vi "Add DAQ Hardware.vi"(7 "Overwrite Existing?":bool=TRUE, 8 "error in (no error)":errorcluster, 9 "Settings":T1={"Name"="", "Description"="", "InputConfiguration"=10078, "TurnOffHWTimedSinglePointAI"=FALSE, "TurnOffHWTimedSinglePointAO"=FALSE, "DAQConversionRateOption"=0, "PortWidth"=8, "Analog Inputs"=[], "Analog Outputs"=[], "DIO Port Settings"=[], "Counter Settings"={"Frequency Measurements"=[], "Period Measurements"=[], "Count Measurements"=[], "Position Measurements"=[]}} {"Counter Settings"."Position Measurements"."ZIndexMode" items=["AHighBHigh"=10040, "AHighBLow"=10041, "ALowBHigh"=10042, "ALowBLow"=10043]; "Counter Settings"."Position Measurements"."Decoding" items=["Decoding1X"=10090, "Decoding2X"=10091, "Decoding4X"=10092, "DecodingPulseCounting"=10313]; "Counter Settings"."Count Measurements"."CountDirection" items=["Down"=10124, "Up"=10128, "ExternallyControlled"=10326]; "Counter Settings"."Count Measurements"."Edge" items=["Falling"=10171, "Rising"=10280]; "Counter Settings"."Period Measurements"."Edge" items=["Falling"=10171, "Rising"=10280]; "Counter Settings"."Frequency Measurements"."Edge" items=["Falling"=10171, "Rising"=10280]; "Analog Outputs"."ChannelType" items=["Voltage", "Current"]; "Analog Inputs"."ChannelType" items=["Voltage", "Current"]; "DAQConversionRateOption" items=["Default", "Maximum"]; "InputConfiguration" items=["NRSE"=10078, "RSE"=10083, "Differential"=10106, "Pseudodifferential"=12529, "Default"=-1]}, 10 "Base Node Path":string="Targets/Controller/Hardware/Chassis/DAQ", 11 "SysDef Ref":T8) -> (0 "error out":errorcluster, 2 "New Node Path":string, 3 "SysDef Ref Out":T8)   [LabVIEW 2019, in "Simple SysDef API.lvlib"]
uses:
  <userlib>/SimpleSysDef/Simple SysDef API.lvlib
  <userlib>/SimpleSysDef/_SubVIs/System Definition Reference.ctl
  NationalInstruments.VeriStand.SystemDefinitionAPI
  <userlib>/SimpleSysDef/_SubVIs/Add DAQ Hardware_Settings.ctl
  <userlib>/SimpleSysDef/_SubVIs/Add DAQ Hardware_Analog Settings.ctl
  <userlib>/SimpleSysDef/_SubVIs/Add DAQ Hardware_Digital Port Settings.ctl
  <userlib>/SimpleSysDef/_SubVIs/Add DAQ Hardware_Digital Settings.ctl
  <userlib>/SimpleSysDef/_SubVIs/Add Frequency Measurement Channels_Settings.ctl
  <userlib>/SimpleSysDef/_SubVIs/Add Count Measurement Channels_Settings.ctl
  <userlib>/SimpleSysDef/_SubVIs/Add Position Measurement Channels_Settings.ctl
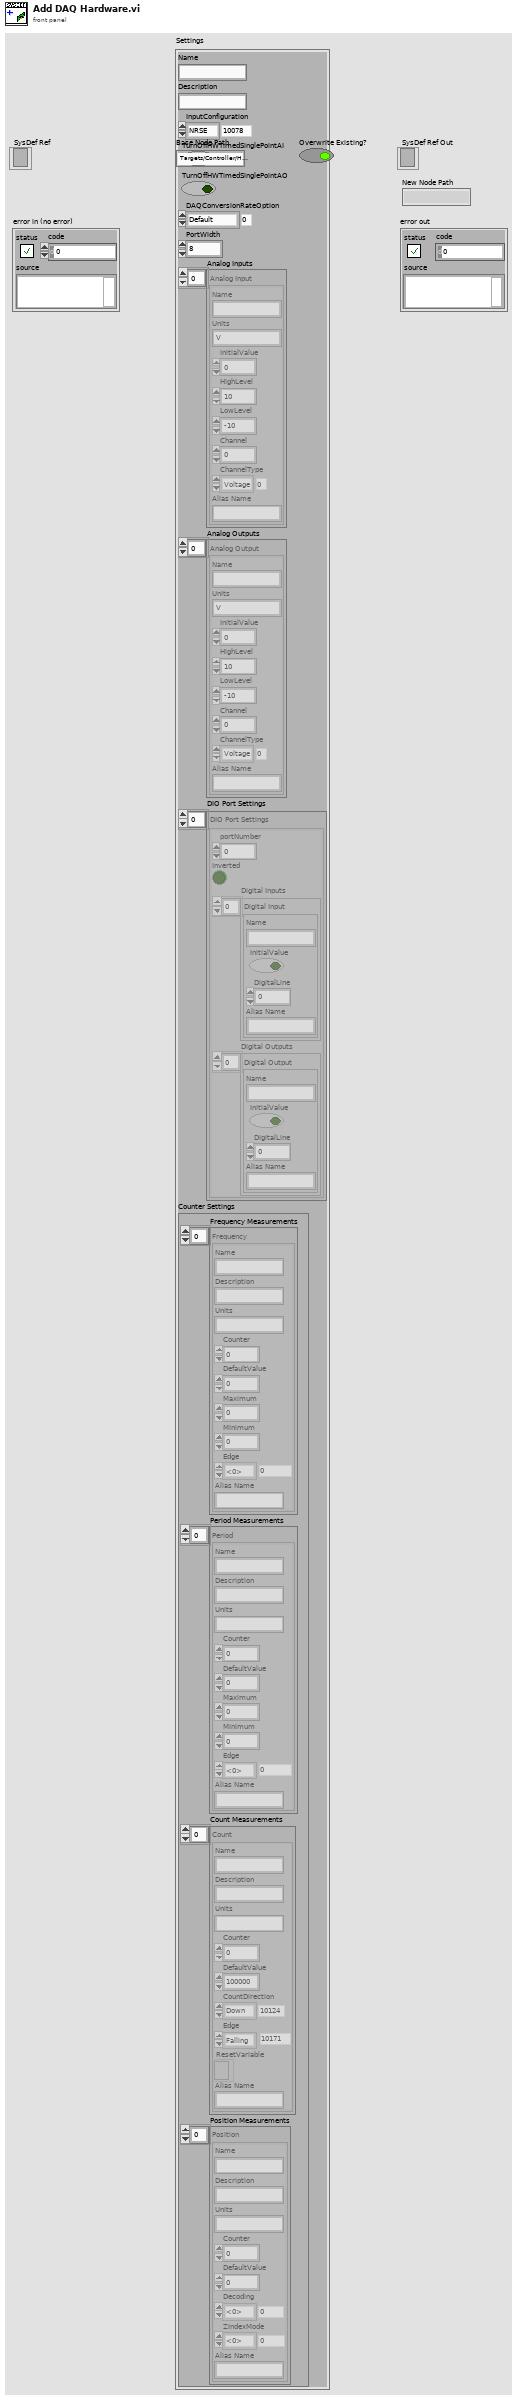
[diagram p1: front panel]
types:
  T1 = typedef "Simple SysDef API.lvlib/Add DAQ Hardware_Settings.ctl" = cluster{"Name":string, "Description":string, "InputConfiguration":i32, "TurnOffHWTimedSinglePointAI":bool, "TurnOffHWTimedSinglePointAO":bool, "DAQConversionRateOption":i32, "PortWidth":u16, "Analog Inputs":T2[], "Analog Outputs":T2[], "DIO Port Settings":T3[], "Counter Settings":cluster{"Frequency Measurements":T5[], "Period Measurements":T5[], "Count Measurements":T6[], "Position Measurements":T7[]}}
  T2 = typedef "Simple SysDef API.lvlib/Add DAQ Hardware_Analog Settings.ctl" = cluster{"Name":string, "Units":string, "InitialValue":dbl, "HighLevel":dbl, "LowLevel":dbl, "Channel":u32, "ChannelType":i32, "Alias Name":string}
  T3 = typedef "Simple SysDef API.lvlib/Add DAQ Hardware_Digital Port Settings.ctl" = cluster{"portNumber":u32, "Inverted":bool, "Digital Inputs":T4[], "Digital Outputs":T4[]}
  T4 = typedef "Simple SysDef API.lvlib/Add DAQ Hardware_Digital Settings.ctl" = cluster{"Name":string, "InitialValue":bool, "DigitalLine":u32, "Alias Name":string}
  T5 = typedef "Simple SysDef API.lvlib/Add Frequency Measurement Channels_Settings.ctl" = cluster{"Name":string, "Description":string, "Units":string, "Counter":u32, "DefaultValue":dbl, "Maximum":dbl, "Minimum":dbl, "Edge":i32, "Alias Name":string}
  T6 = typedef "Simple SysDef API.lvlib/Add Count Measurement Channels_Settings.ctl" = cluster{"Name":string, "Description":string, "Units":string, "Counter":u32, "DefaultValue":dbl, "CountDirection":i32, "Edge":i32, "ResetVariable":refnum<k24>, "Alias Name":string}
  T7 = typedef "Simple SysDef API.lvlib/Add Position Measurement Channels_Settings.ctl" = cluster{"Name":string, "Description":string, "Units":string, "Counter":u32, "DefaultValue":dbl, "Decoding":i32, "ZIndexMode":i32, "Alias Name":string}
  T8 = typedef "Simple SysDef API.lvlib/System Definition Reference.ctl" = refnum<k24>
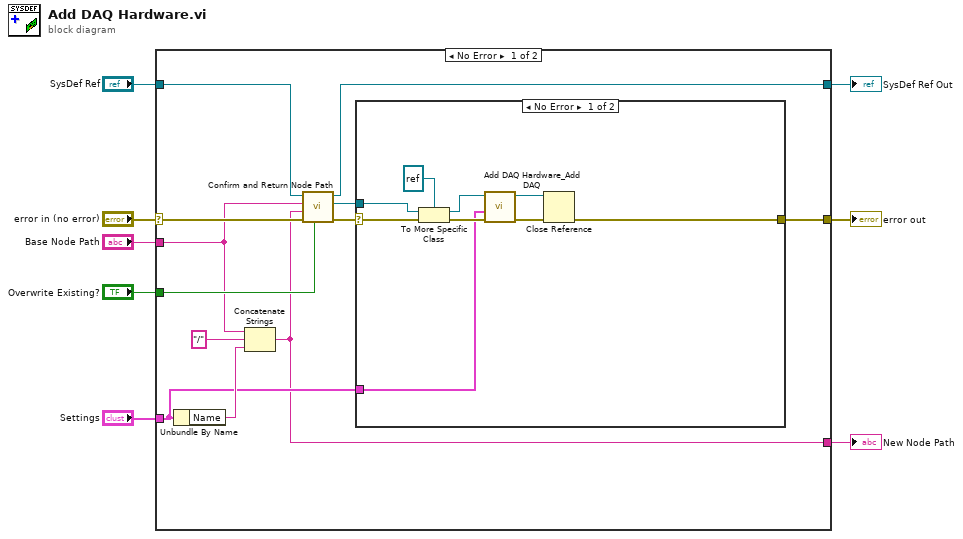
[diagram p0: block diagram]
diagram:
  n1 = case shown="No Error" "error in (no error)" {
    selector: "error in (no error)" -> [w20 w32]
    tunnel: [w16 w32] -> w7
    tunnel: "SysDef Ref" -> [w19 w31]
    tunnel: [w9 w31] -> w5
    tunnel: "Base Node Path" -> [w11 _]
    tunnel: "Overwrite Existing?" -> [w13 _]
    tunnel: "Settings" -> [w12 _]
    tunnel: [w10 _] -> w1
    frame No Error {
      n2 = Unbundle By Name(w12) -> ("Name"=w17:string)
      n3 = Concatenate Strings(w11, "/" ("string"), w17) -> (w10:string)
      n4 = call <userlib>:"Confirm and Return Node Path.vi"("Overwrite Existing?"=w13, "error in (no error)"=w20, "New Node Path"=w10, "Base Node Path"=w11, "SysDef Ref"=w19) -> ("error out"=w14:errorcluster, "Node Ref"=w15:refnum<k24>, "SysDef Ref Out"=w9:T8)  [unwired: 4 in]
      n5 = case shown="No Error" w14 {
        selector: w14 -> [w28 w30]
        tunnel: [w21 w30] -> w16
        tunnel: w15 -> [w29 _]
        tunnel: w12 -> [w24 _]
        frame No Error {
          n6 = To More Specific Class(target class=refnum<k24> refnum ("Node Ref"), reference=w29, error in=w28) -> (specific class reference=w26:refnum<k24>, error out=w25:errorcluster)
          n7 = call <userlib>:"Add DAQ Hardware_Add DAQ.vi"("error in (no error)"=w25, "Settings"=w24, "DAQ Ref"=w26) -> ("error out"=w22:errorcluster, "DAQ Ref Out"=w23:refnum<k24>)  [unwired: 7 in]
          n8 = Close Reference(reference=w23, error in (no error)=w22) -> (error out=w21:errorcluster)
        }
        frame Error {
        }
      }
    }
    frame Error {
    }
  }
  "SysDef Ref Out" <- w5
  "error out" <- w7
  "New Node Path" <- w1
